vi "Update_inventario.vi"(8 "error in (no error)":errorcluster, 9 "Inventario":dbl, 10 "Index":i32, 11 "Nestle_Actor in":refnum<class "Nestle_Actor.lvclass">) -> (0 "error out":errorcluster, 3 "Nestle_Actor out":refnum<class "Nestle_Actor.lvclass">)   [LabVIEW 2019, in "Nestle_Actor.lvlib" / "Nestle_Actor.lvclass"]
uses:
  Nestle_Actor.lvclass
  Nestle_Actor.lvclass/Nestle_Actor.ctl
  <vilib>/Utility/config.llb/Write Key (String).vi
  <vilib>/Utility/config.llb/NI_LVConfig.lvlib
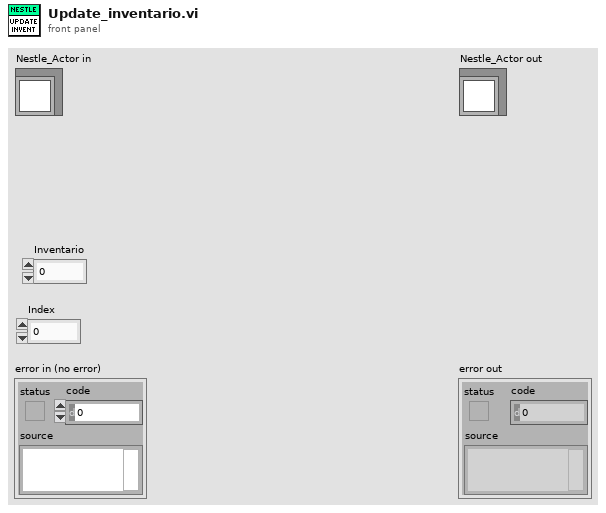
[diagram p1: front panel]
types:
  T1 = typedef "NI_LVConfig.lvlib/Config Data RefNum.ctl" = refnum<k1>
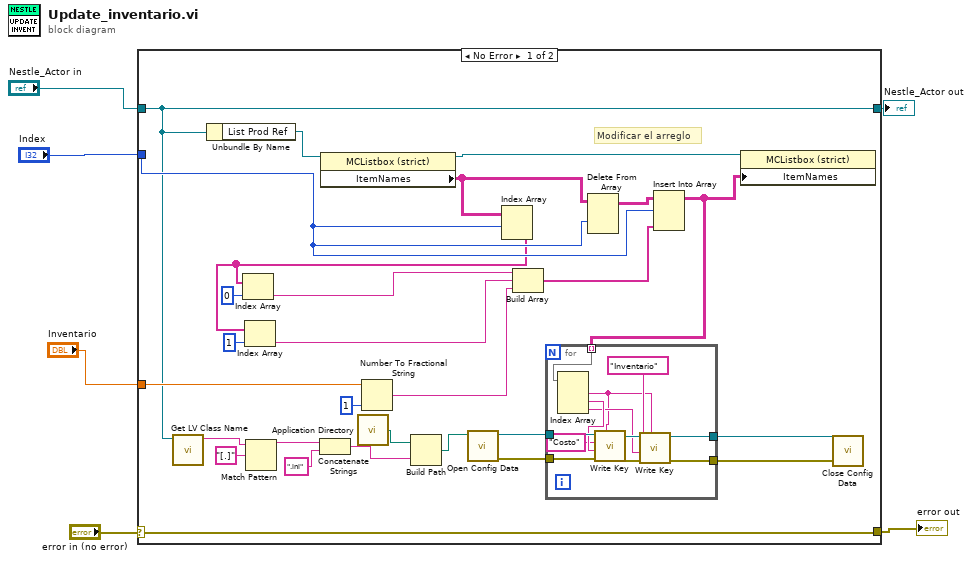
[diagram p0: block diagram]
diagram:
  n1 = case shown="No Error" "error in (no error)" {
    selector: "error in (no error)" -> [w34 w48]
    tunnel: [w34 w48] -> w5
    tunnel: [w24 w47] -> w3
    tunnel: "Nestle_Actor in" -> [w24 w47]
    tunnel: "Index" -> [w29 _]
    tunnel: "Inventario" -> [w26 _]
    frame No Error {
      # "Modificar el arreglo"
      n2 = call <vilib>:"Get LV Class Name.vi"("object"=w24) -> ("class name"=w22:string)  [unwired: 9 in, 1 out]
      n3 = Unbundle By Name(w24) -> ("List Prod Ref"=w30:refnum<vi>)
      n4 = Match Pattern(string=w22, regular expression="[.]") -> (before substring=w21:string)  [unwired: 1 in, 3 out]
      n5 = Concatenate Strings(w21, ".ini" ("string")) -> (w18:string)
      n6 = property class="MCListbox (strict)"(reference=w30) -> (reference out=w32:refnum<vi>, "ItemNames"=w33:string[][])  [unwired: 1 in, 1 out]
      n7 = call <vilib>:"Application Directory.vi"() -> ("Application Directory"=w19:path)
      n8 = Number To Fractional String(number=w26, precision (6)=i16 1) -> (F-format string=w27:string)  [unwired: 2 in]
      n9 = Build Path(base path=w19, name or relative path=w18) -> (appended path=w17:path)
      n10 = call <vilib>:"Open Config Data.vi"("configuration file path"=w17) -> ("error out"=w15:errorcluster, "refnum"=w16:T1)  [unwired: 8 in, 1 out]
      n11 = Index Array(array=w33, index (row)=w29) -> (element=w10:string[])  [unwired: 1 in]
      n12 = Index Array(array=w10, index=0) -> (element=w7:string)
      n13 = Index Array(array=w10, index=1) -> (element=w8:string)
      n14 = Build Array(w7, w8, w27) -> (w25:string[])
      n15 = Delete From Array(array=w33, index (row)=w29) -> (array with subset deleted=w31:string[][])  [unwired: 2 in, 1 out]
      n16 = Insert Into Array(array=w31, index (row)=w29, new element=w25) -> (w14:string[][])  [unwired: 1 in]
      n17 = for {
        tunnel: w16 -> [w44]
        tunnel: w15 -> [w43]
        tunnel: w14 -> [w38] mode=indexing
        tunnel: [w36] -> w13
        tunnel: [w35] -> w12
        n18 = Index Array(array=w38) -> (element #1=w37:string, element #2=w42:string, element #3=w41:string)  [unwired: 3 in]
        n19 = call-poly <vilib>:"Write Key.vi"("section"=w37, "error in (no error)"=w43, "value"=w42, "key"="Costo", "refnum"=w44) -> ("error out"=w45:errorcluster, "refnum out"=w46:T1)  [unwired: 4 in, 1 out]
        n20 = call-poly <vilib>:"Write Key.vi"("section"=w37, "error in (no error)"=w45, "value"=w41, "key"="Inventario", "refnum"=w46) -> ("error out"=w36:errorcluster, "refnum out"=w35:T1)  [unwired: 4 in, 1 out]
      }
      n21 = property class="MCListbox (strict)"(reference=w32, "ItemNames"=w14) -> ()  [unwired: 1 in, 2 out]
      n22 = call <vilib>:"Close Config Data.vi"("error in (no error)"=w13, "refnum"=w12) -> ()  [unwired: 8 in, 2 out]
    }
    frame Error {
    }
  }
  "error out" <- w5
  "Nestle_Actor out" <- w3
